vi "Servo.vi"(0 "Servo 4":u32(slide) scale=500.0..2250.0, 1 "Servo 3":u32(slide) scale=500.0..2250.0, 2 "Servo 2":u32(slide) scale=500.0..2250.0, 3 "Servo 1":u32(slide) scale=500.0..2250.0) -> ()   [LabVIEW 2015]
uses:
  <vilib>/rvi/eio/common/nirviEmuTemplateMethod_errors.vi
  <vilib>/eio/EIONode/EIONode.xnode
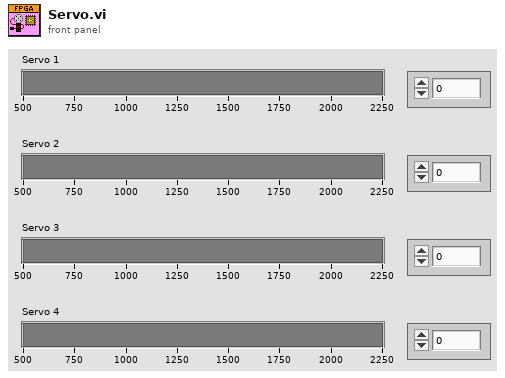
[diagram p1: front panel]
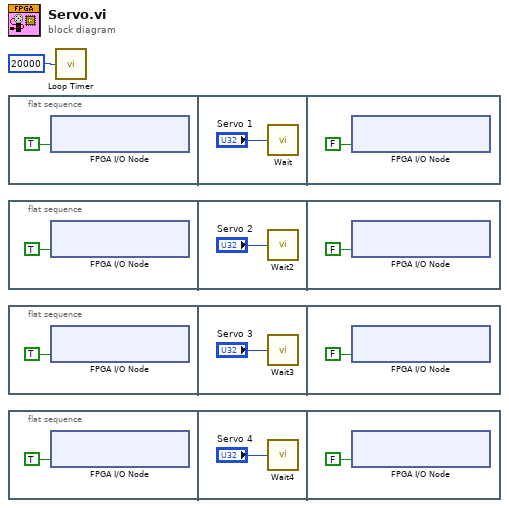
[diagram p0: block diagram]
diagram:
  n1 = flat-sequence {
    frame #0 {
      n2 = xnode "FPGA I/O Node"("ConnectorC/DIO0"=TRUE) -> ()  [unwired: 1 in, 1 out]
    }
    frame #1 {
      n3 = call "Wait"("Count(uSec)"="Servo 1") -> ()  [unwired: 1 out]
    }
    frame #2 {
      n4 = xnode "FPGA I/O Node"("ConnectorC/DIO0"=FALSE) -> ()  [unwired: 1 in, 1 out]
    }
  }
  n5 = flat-sequence {
    frame #0 {
      n6 = xnode "FPGA I/O Node"("ConnectorC/DIO1"=TRUE) -> ()  [unwired: 1 in, 1 out]
    }
    frame #1 {
      n7 = call "Wait2"("Count(uSec)"="Servo 2") -> ()  [unwired: 1 out]
    }
    frame #2 {
      n8 = xnode "FPGA I/O Node"("ConnectorC/DIO1"=FALSE) -> ()  [unwired: 1 in, 1 out]
    }
  }
  n9 = flat-sequence {
    frame #0 {
      n10 = xnode "FPGA I/O Node"("ConnectorC/DIO2"=TRUE) -> ()  [unwired: 1 in, 1 out]
    }
    frame #1 {
      n11 = call "Wait3"("Count(uSec)"="Servo 3") -> ()  [unwired: 1 out]
    }
    frame #2 {
      n12 = xnode "FPGA I/O Node"("ConnectorC/DIO2"=FALSE) -> ()  [unwired: 1 in, 1 out]
    }
  }
  n13 = flat-sequence {
    frame #0 {
      n14 = xnode "FPGA I/O Node"("ConnectorC/DIO3"=TRUE) -> ()  [unwired: 1 in, 1 out]
    }
    frame #1 {
      n15 = call "Wait4"("Count(uSec)"="Servo 4") -> ()  [unwired: 1 out]
    }
    frame #2 {
      n16 = xnode "FPGA I/O Node"("ConnectorC/DIO3"=FALSE) -> ()  [unwired: 1 in, 1 out]
    }
  }
  n17 = call "Loop Timer"("Count(uSec)"=u32 20000) -> ()  [unwired: 1 out]
